vi "Commands array generator.vi"(4 "Axis 1":string, 5 "Heigth":i32, 6 "Axis in":string, 7 "Width":i32, 8 "Axes speed \n(µm/s)":i32, 9 "Y Step size in µm":i32, 10 "T/F product array":bool[][](array[boolean]), 11 "Space defined array":dbl[][](array[numeric])) -> (2 "Command Array":string[][](array[string]), 3 "Time Array":dbl[][](array[numeric]))   [LabVIEW 2016]
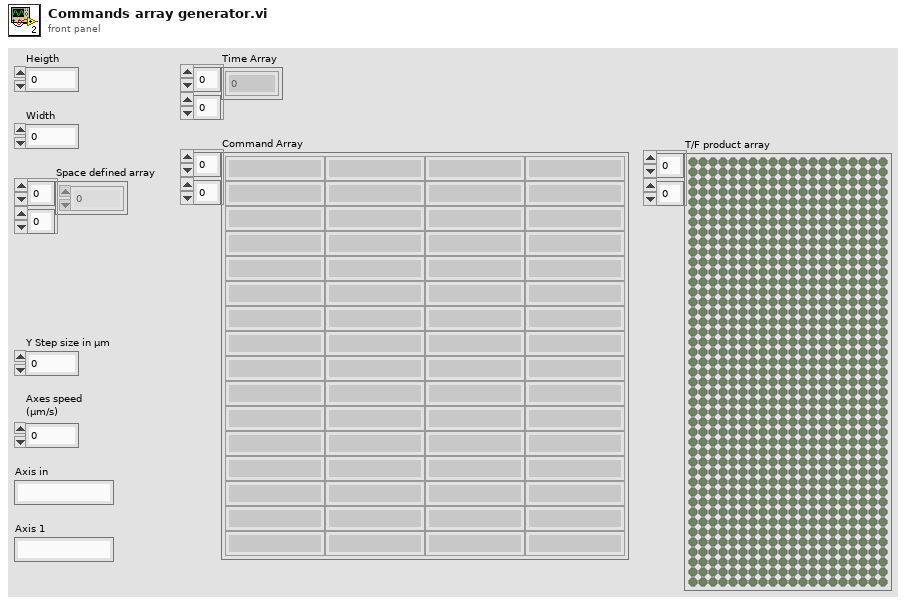
[diagram p1: front panel]
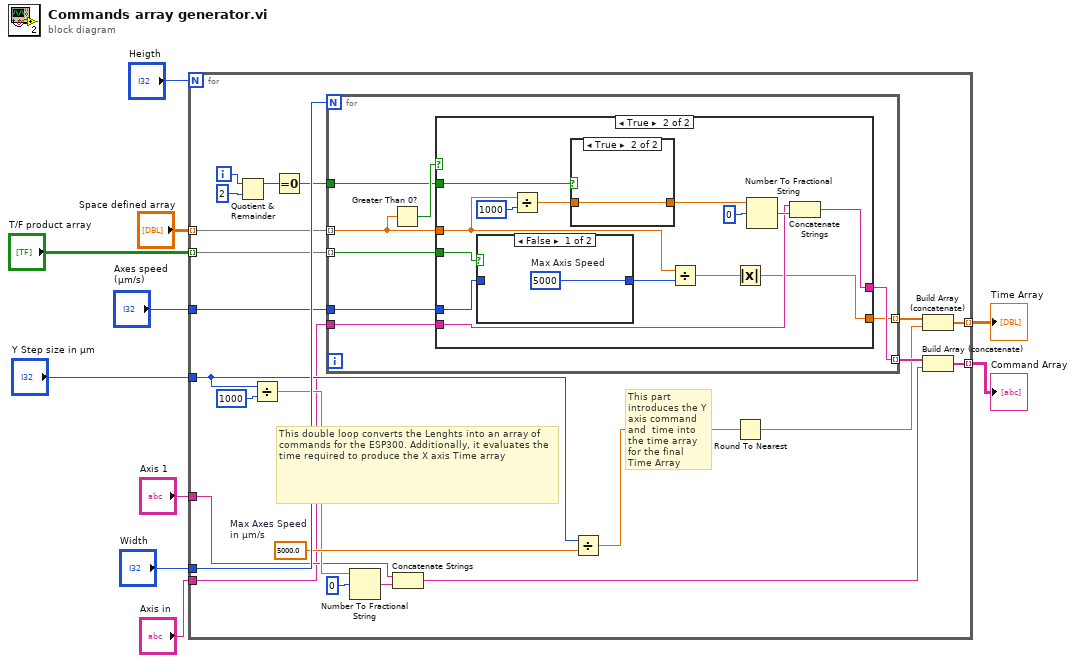
[diagram p0: block diagram]
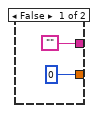
[diagram p2: hidden frame]
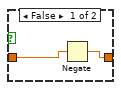
[diagram p4: hidden frame]
diagram:
  n1 = for {
    N: "Heigth" -> [_]
    tunnel: "Width" -> [w33]
    tunnel: "Space defined array" -> [w32] mode=indexing
    tunnel: [w29] -> w5 mode=indexing
    tunnel: "T/F product array" -> [w22] mode=indexing
    tunnel: [w19] -> w6 mode=indexing
    tunnel: "Y Step size in µm" -> [w14]
    tunnel: "Axis 1" -> [w13]
    tunnel: "Axis in" -> [w12]
    tunnel: "Axes speed \n(µm/s)" -> [w11]
    i -> [w24]
    w18 = 5000.0  # Max Axes Speed in µm/s
    # "This part introduces the Y axis command and  time into the time array for the final Time Array"
    # "This double loop converts the Lenghts into an array of commands for the ESP300. Additionally, it evaluates the time required to produce the X axis Time array"
    n2 = Quotient & Remainder(x=w24, y=2) -> (x-y*floor(x/y)=w26:i32)  [unwired: 1 out]
    n3 = Divide(x=w14, y=1000) -> (x/y=w17:dbl)
    n4 = Equal To 0?(x=w26) -> (x = 0?=w23:bool)
    n5 = for {
      N: w33 -> [_]
      tunnel: w32 -> [w41] mode=indexing
      tunnel: [w39] -> w28 mode=indexing
      tunnel: w23 -> [w38]
      tunnel: [w37] -> w20 mode=indexing
      tunnel: w22 -> [w36] mode=indexing
      tunnel: w12 -> [w35]
      tunnel: w11 -> [w34]
      n6 = Greater Than 0?(x=w41) -> (x > 0?=w40:bool)
      n7 = case shown="True" w40 {
        tunnel: w41 -> [_ w51]
        tunnel: ["" w56] -> w39
        tunnel: w38 -> [_ w54]
        tunnel: [0 w44] -> w37
        tunnel: w36 -> [_ w49]
        tunnel: w35 -> [_ w46]
        tunnel: w34 -> [_ w45]
        frame False {
        }
        frame True {
          n8 = case shown="False" w49 {
            tunnel: [w58 w59] -> w50
            tunnel: w45 -> [_ w59]
            frame False {
              w58 = 5000  # Max Axis Speed
            }
            frame True {
            }
          }
          n9 = Divide(x=w51, y=1000) -> (x/y=w52:dbl)
          n10 = case shown="True" w54 {
            tunnel: w52 -> [w61 w62]
            tunnel: [w60 w62] -> w53
            frame False {
              n11 = Negate(x=w61) -> (-x=w60:dbl)
            }
            frame True {
            }
          }
          n12 = Divide(x=w51, y=w50) -> (x/y=w47:dbl)
          n13 = Absolute Value(x=w47) -> (abs(x)=w44:dbl)
          n14 = Number To Fractional String(number=w53, width (-)=i16 0) -> (F-format string=w48:string)  [unwired: 2 in]
          n15 = Concatenate Strings(w46, w48) -> (w56:string)
        }
      }
    }
    n16 = Number To Fractional String(number=w17, width (-)=i16 0) -> (F-format string=w21:string)  [unwired: 2 in]
    n17 = Concatenate Strings(w13, w21) -> (w30:string)
    n18 = Divide(x=w14, y=w18) -> (x/y=w16:dbl)
    n19 = Round To Nearest(number=w16) -> (nearest integer value=w15:dbl)
    n20 = Build Array (concatenate)(w20, w15) -> (w19:dbl[])
    n21 = Build Array (concatenate)(w28, w30) -> (w29:string[])
  }
  "Time Array" <- w6
  "Command Array" <- w5
